vi "Close.vi"(8 "error in (no error)":errorcluster, 11 "Hioki BT4560B in":refnum<class "Hioki BT4560B.lvclass">) -> (0 "error out":errorcluster, 3 "Hioki BT4560B out":refnum<class "Hioki BT4560B.lvclass">)   [LabVIEW 2021, in "Concrete.lvlib" / "Hioki BT4560B.lvclass"]
uses:
  Hioki BT4560B.lvclass
  Hioki BT4560B.lvclass/Hioki BT4560B.ctl
  Harware Abstraction/ACIR/ACIR.lvclass
  <instrlib>/HIOKI BT4560/HIOKI BT4560.lvlib
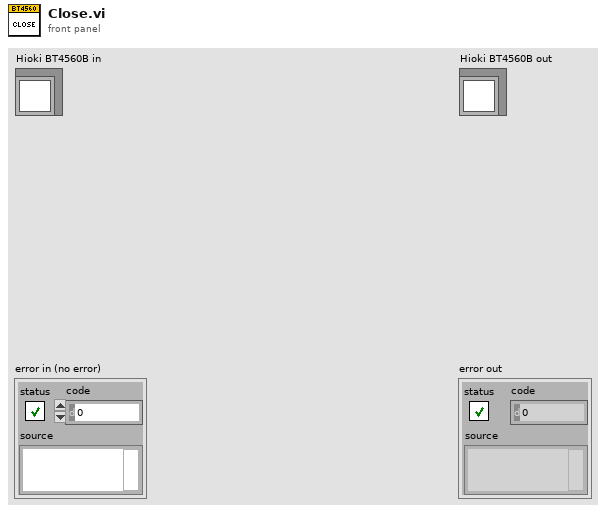
[diagram p1: front panel]
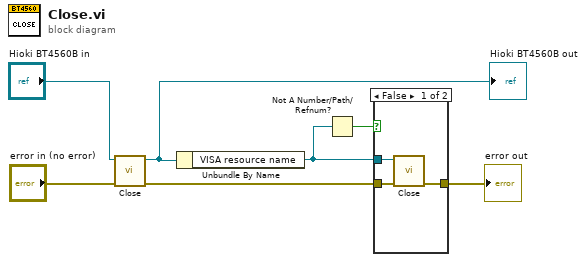
[diagram p0: block diagram]
diagram:
  n1 = call-parent <instrlib>:"Close.vi"("error in (no error)"="error in (no error)", "Instrument in"="Hioki BT4560B in") -> ("error out"=w5:errorcluster, "Instrument out"=w3:refnum<class "Hioki BT4560B.lvclass">)  [unwired: 8 in]
  "Hioki BT4560B out" <- w3
  n2 = Unbundle By Name(w3) -> ("VISA resource name"=w2:refnum<visa-resource-name>)
  n3 = Not A Number/Path/Refnum?(number/path/refnum=w2) -> (NaN/Path/Refnum?=w1:bool)
  n4 = case shown="False" w1 {
    tunnel: w5 -> [w10 w11]
    tunnel: [w9 w11] -> w4
    tunnel: w2 -> [w8 _]
    frame False {
      n5 = call <instrlib>:"Close.vi"("error in (no error)"=w10, "VISA resource name"=w8) -> ("error out"=w9:errorcluster)  [unwired: 9 in]
    }
    frame True {
    }
  }
  "error out" <- w4
